vi "MAV_CMD_MISSION_START.vi"(11 "Target System and Target Component":u8=1) -> (3 "MAVLink Message":u8[](array[numeric]))   [LabVIEW 2014]
panel:
  out "Payload Size":i32
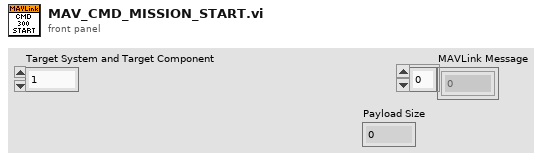
[diagram p1: front panel]
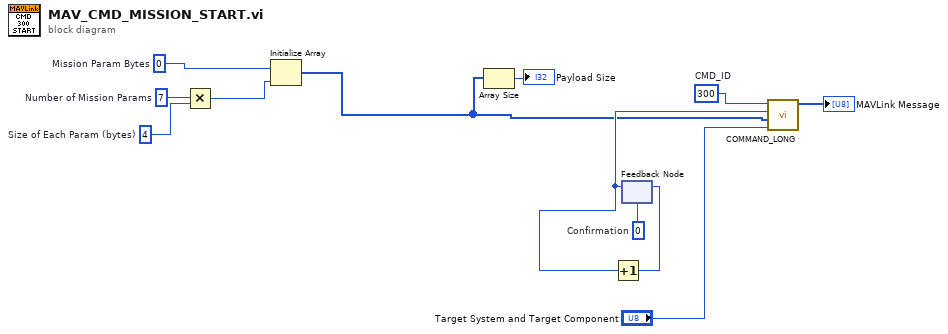
[diagram p0: block diagram]
diagram:
  w7 = u8 0  # Confirmation
  w10 = 4  # Size of Each Param (bytes)
  w11 = 7  # Number of Mission Params
  w12 = u8 0  # Mission Param Bytes
  w5 = u16 300  # CMD_ID
  n1 = Multiply(x=w11, y=w10) -> (x*y=w9:i32)
  n2 = Initialize Array(w12, w9) -> (w2:u8[])
  n3 = Array Size(array=w2) -> (size(s)=→"Payload Size":i32)
  n4 = feedback #1(w7) -> (w4:u8)
  n5 = Increment(x=w4) -> (x+1=w6:u8)
  n6 = feedback-in #1(w6) -> ()
  n7 = call "COMMAND_LONG.vi"("Target System and Target Component"="Target System and Target Component", "Mission Params"=w2, "Confirmation"=w4, "Command ID"=w5) -> ("MAVLink Message"=→"MAVLink Message":u8[])  [unwired: 7 in]
